vi "Droplet Size.vi"(10 "Flow Rate":dbl, 11 "Array":dbl[](array[numeric])) -> (3 "droplet size":dbl)   [LabVIEW 2020]
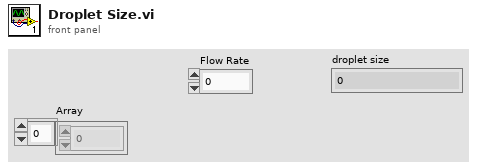
[diagram p1: front panel]
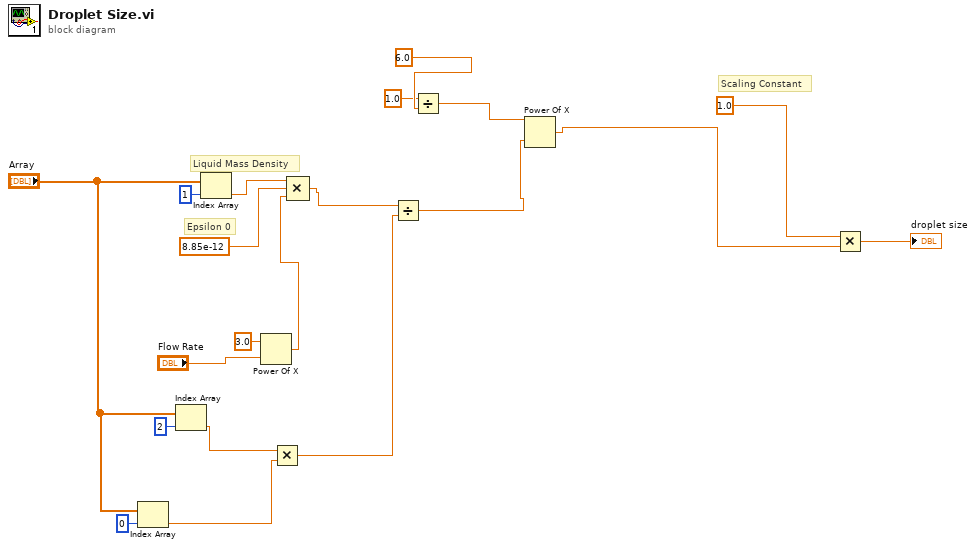
[diagram p0: block diagram]
diagram:
  # "Epsilon 0"
  # "Liquid Mass Density"
  # "Scaling Constant"
  n1 = Index Array(array="Array", index=0) -> (element=w9:dbl)
  n2 = Index Array(array="Array", index=2) -> (element=w11:dbl)
  n3 = Index Array(array="Array", index=1) -> (element=w18:dbl)
  n4 = Power Of X(1:"Flow Rate", 2:3.0 ("y")) -> (0:w14:dbl)
  n5 = Multiply(x=w11, y=w9) -> (x*y=w8:dbl)
  n6 = Compound Arithmetic op=MULTIPLY(w18, 8.85e-12 ("y"), w14) -> (w13:dbl)
  n7 = Divide(x=w13, y=w8) -> (x/y=w5:dbl)
  n8 = Divide(x=1.0, y=6.0) -> (x/y=w2:dbl)
  n9 = Power Of X(1:w5, 2:w2) -> (0:w1:dbl)
  n10 = Multiply(x=1.0, y=w1) -> (x*y=→"droplet size":dbl)
